vi "dfd_DFXP Add (ss).vi"(5 "quantize output? (T)":bool=TRUE, 7 "op params":T5={"source"=0, "is floating?"=FALSE, "o-mode"=enum."Wrap", "q-mode"=enum."Truncation", "wl"=1, "high limit"=0, "low limit"=0, "iwl"=0, "sign?"=TRUE} {"source" items=["Coef a/k"=0, "Coef b/v"=7, "Input"=1, "Output"=2, "Multiplicand"=3, "Product"=4, "Sum"=5, "Delay"=6, "Gain"=8]}, 8 "filtering statistics in":T4(array[cluster]) {"statistics information"."min value" format="%.2f"; "statistics information"."max value" format="%.2f"; "Quantizer Source" items=["Coefficients a/k"=0, "Coefficients b/v"=7, "Input"=1, "Output"=2, "Multiplicand"=3, "Product"=4, "Sum"=5, "Delay"=6]}, 9 "Value in 2":T1={"value"=0, "wl"=0, "iwl"=0, "Signed"=TRUE} {"value" format="%.0x"}, 11 "Value in":T1={"value"=0, "wl"=0, "iwl"=0, "Signed"=TRUE} {"value" format="%.0x"}) -> (0 "filtering statistics out":T4(array[cluster]) {"statistics information"."min value" format="%.2f"; "statistics information"."max value" format="%.2f"; "Quantizer Source" items=["Coefficients a/k"=0, "Coefficients b/v"=7, "Input"=1, "Output"=2, "Multiplicand"=3, "Product"=4, "Sum"=5, "Delay"=6]}, 3 "Value out":T1={"value"=0, "wl"=0, "iwl"=0, "Signed"=TRUE} {"value" format="%.0x"})   [LabVIEW 2017, in "NI_DigFilter_FXP.lvlib"]
uses:
  <vilib>/addons/Digital Filter Design/NI_DigFilter_FXP.lvlib
  <vilib>/addons/Digital Filter Design/_Objects.llb/dfd_DFXP Data Type (scaler).ctl
  <vilib>/addons/Digital Filter Design/_Objects.llb/dfd_DFXP Data Type 128bits (scaler).ctl
  <vilib>/addons/Digital Filter Design/_Objects.llb/dfd_DFXP Operation Parameter.ctl
  <vilib>/addons/Digital Filter Design/_Objects.llb/dfd_Internal Quantization Srcs.ctl
  <vilib>/addons/Digital Filter Design/_Objects.llb/DFD Quantization Sources.ctl
  <vilib>/addons/Digital Filter Design/_Objects.llb/DFD FXP Statistics Data.ctl
  <vilib>/addons/Digital Filter Design/NI_DigFilterLicensed.lvlib
panel:
  in  "Value type64":T1={"value"=0, "wl"=0, "iwl"=0, "Signed"=TRUE} {"value" format="%.0x"}
  in  "Value type":T1={"value"=0, "wl"=0, "iwl"=0, "Signed"=TRUE} {"value" format="%.0x"}
  in  "Value type":T7 {"Low 64" format="%.0x"; "High 64" format="%.0x"}
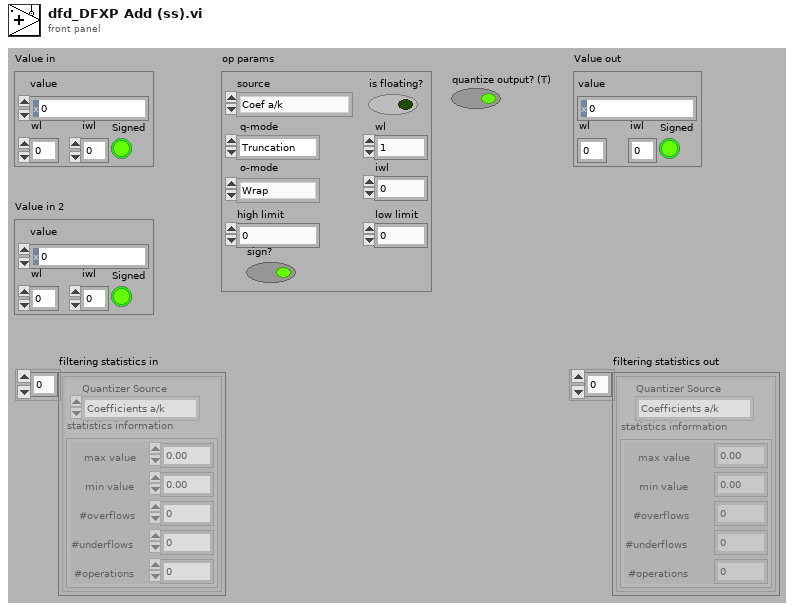
[diagram p1: front panel]
types:
  T1 = typedef "dfd_DFXP Data Type (scaler).ctl" = cluster{"value":i64, "wl":i16, "iwl":i16, "Signed":bool}
  T2 = typedef "NI_DigFilterLicensed.lvlib/DFD Quantization Sources.ctl" = u16
  T3 = typedef "NI_DigFilterLicensed.lvlib/DFD FXP Statistics Data.ctl" = cluster{"max value":ext, "min value":ext, "#overflows":i32, "#underflows":i32, "#operations":i32}
  T4 = cluster{"Quantizer Source":T2, "statistics information":T3}[]
  T5 = typedef "dfd_DFXP Operation Parameter.ctl" = cluster{"source":T6, "is floating?":bool, "o-mode":enum16{"Saturation", "Wrap"}, "q-mode":enum16{"Nearest", "Truncation"}, "wl":i16, "high limit":i64, "low limit":i64, "iwl":i16, "sign?":bool}
  T6 = typedef "NI_DigFilterLicensed.lvlib/dfd_Internal Quantization Srcs.ctl" = u16
  T7 = typedef "dfd_DFXP Data Type 128bits (scaler).ctl" = cluster{"Low 64":u64, "High 64":i64, "wl":i16, "iwl":i16}
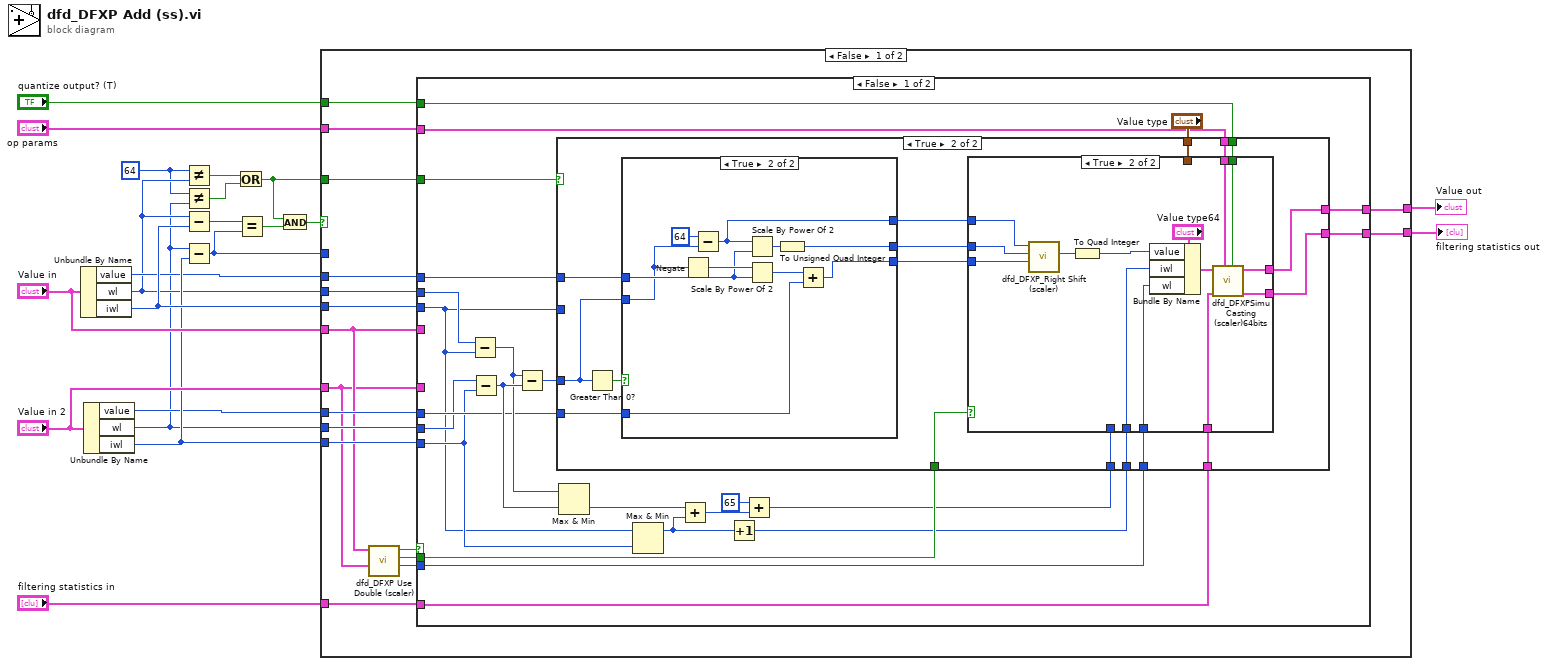
[diagram p0: block diagram]
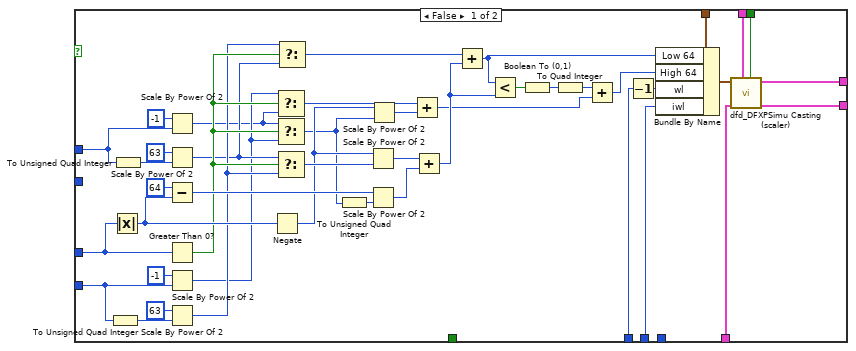
[diagram p2: hidden frame]
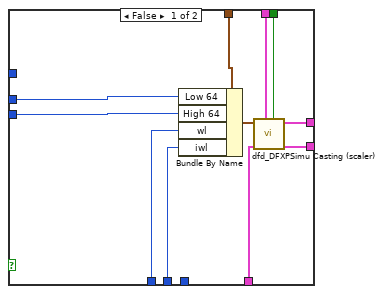
[diagram p3: hidden frame]
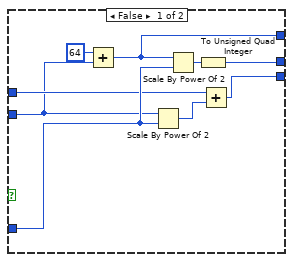
[diagram p4: hidden frame]
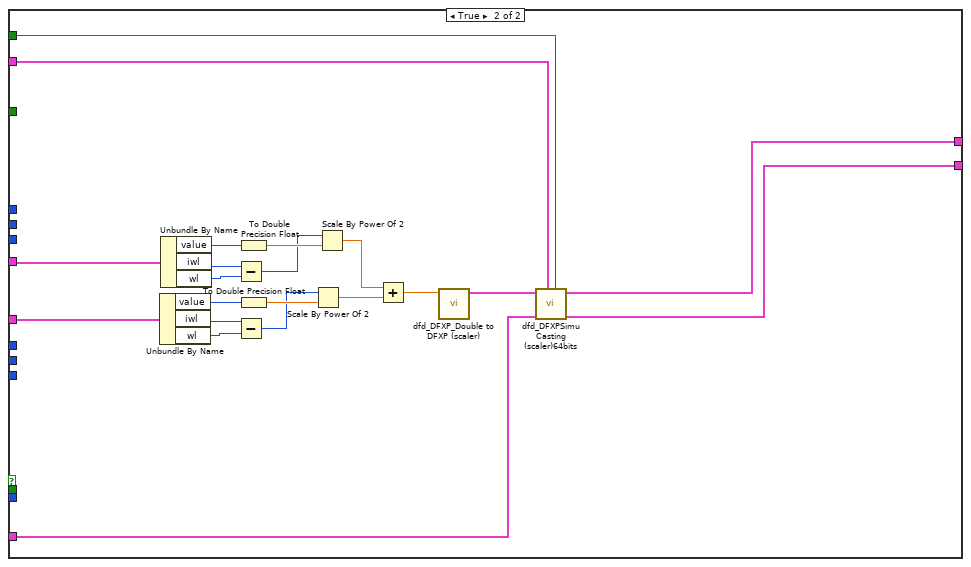
[diagram p5: hidden frame]
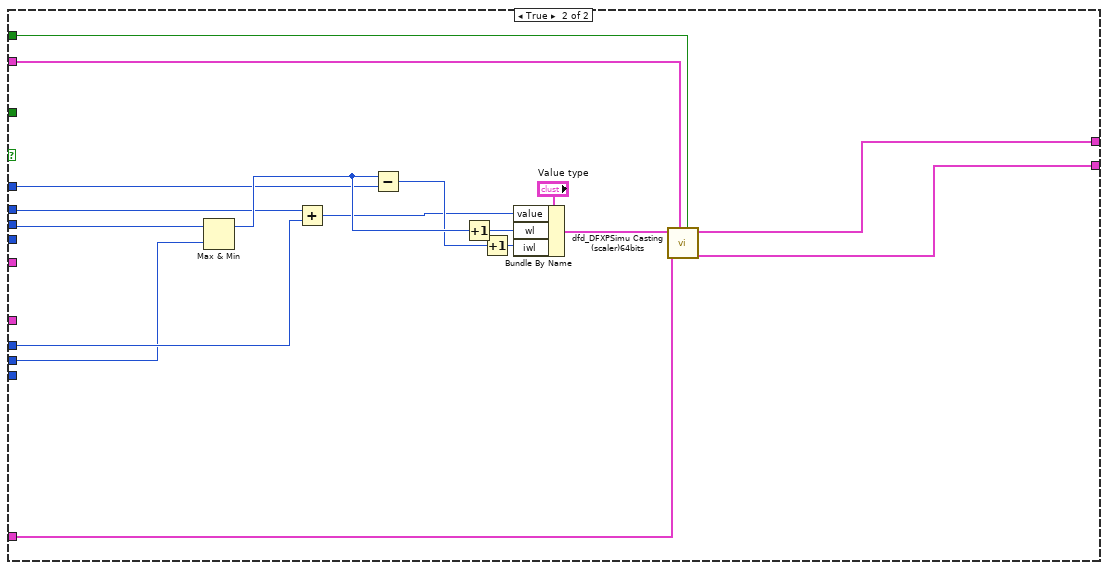
[diagram p6: hidden frame]
diagram:
  w3 = i16 64 ("y")
  n1 = Unbundle By Name("Value in") -> ("value"=w12:i64, "wl"=w5:i16, "iwl"=w16:i16)
  n2 = Unbundle By Name("Value in 2") -> ("value"=w11:i64, "wl"=w4:i16, "iwl"=w15:i16)
  n3 = Not Equal?(x=w3, y=w5) -> (x != y?=w6:bool)
  n4 = Not Equal?(x=w3, y=w4) -> (x != y?=w2:bool)
  n5 = Subtract(x=w5, y=w16) -> (x-y=w10:i16)
  n6 = Subtract(x=w4, y=w15) -> (x-y=w9:i16)
  n7 = Or(x=w6, y=w2) -> (x .or. y?=w1:bool)
  n8 = Equal?(x=w10, y=w9) -> (x = y?=w8:bool)
  n9 = And(x=w1, y=w8) -> (x .and. y?=w7:bool)
  n10 = case shown="False" w7 {
    tunnel: w5 -> [w35 w193]
    tunnel: w16 -> [w34 _]
    tunnel: w4 -> [w32 w191]
    tunnel: w15 -> [w31 _]
    tunnel: w11 -> [w33 w192]
    tunnel: w12 -> [w36 w194]
    tunnel: "Value in" -> [w26 _]
    tunnel: "Value in 2" -> [w25 _]
    tunnel: "filtering statistics in" -> [w30 w190]
    tunnel: "op params" -> [w37 w196]
    tunnel: [w28 w188] -> w18
    tunnel: [w29 w189] -> w19
    tunnel: "quantize output? (T)" -> [w38 w197]
    tunnel: w9 -> [_ w195]
    tunnel: w1 -> [w27 _]
    frame False {
      n11 = call <vilib>:"dfd_DFXP Use Double (scaler).vi"("Value in 2"=w25, "Value in"=w26) -> ("Result wl"=w22:i16, "Use 64?"=w23:bool, "Use double?"=w24:bool)  [unwired: 7 out]
      n12 = case shown="False" w24 {
        tunnel: [w45 w183] -> w28
        tunnel: w30 -> [w46 w185]
        tunnel: [w44 w184] -> w29
        tunnel: w37 -> [w43 w182]
        tunnel: w36 -> [w56 _]
        tunnel: w35 -> [w55 _]
        tunnel: w34 -> [w39 _]
        tunnel: w33 -> [w54 _]
        tunnel: w32 -> [w53 _]
        tunnel: w31 -> [w52 _]
        tunnel: w38 -> [w42 w181]
        tunnel: w26 -> [_ w177]
        tunnel: w25 -> [_ w172]
        tunnel: w27 -> [w51 _]
        tunnel: w23 -> [w50 _]
        tunnel: w22 -> [w40 _]
        frame False {
          n13 = Subtract(x=w55, y=w39) -> (x-y=w58:i16)
          n14 = Subtract(x=w53, y=w52) -> (x-y=w62:i16)
          n15 = Subtract(x=w58, y=w62) -> (x-y=w41:i16)
          n16 = Max & Min(x=w58, y=w62) -> (min(x,y)=w61:i16)  [unwired: 1 out]
          n17 = Max & Min(x=w39, y=w52) -> (max(x,y)=w57:i16)  [unwired: 1 out]
          n18 = Add(x=w61, y=w57) -> (x+y=w60:i16)
          n19 = Increment(x=w57) -> (x+1=w47:i16)
          n20 = Add(x=i16 65, y=w60) -> (x+y=w48:i16)
          n21 = case shown="True" w51 {
            tunnel: w41 -> [w76 w119]
            tunnel: w56 -> [w75 w121]
            tunnel: w54 -> [w77 w120]
            tunnel: w50 -> [_ w116]
            tunnel: "Value type" -> [w69 w115]
            tunnel: w48 -> [w71 w114]
            tunnel: w47 -> [w70 w113]
            tunnel: w46 -> [w68 w112]
            tunnel: [w64 w111] -> w45
            tunnel: [w65 w110] -> w44
            tunnel: w43 -> [w67 w109]
            tunnel: w42 -> [w66 w108]
            tunnel: w40 -> [_ w106]
            tunnel: w39 -> [_ _]
            frame False {
              n22 = To Unsigned Quad Integer(1:w77) -> (0:w100:u64)
              n23 = Absolute Value(x=w76) -> (abs(x)=w97:i16)
              n24 = To Unsigned Quad Integer(1:w75) -> (0:w101:u64)
              n25 = Scale By Power Of 2(n=-1, x=w75) -> (x*2^n=w78:i64)
              n26 = Scale By Power Of 2(n=63, x=w101) -> (x*2^n=w89:u64)
              n27 = Subtract(x=i16 64, y=w97) -> (x-y=w104:i16)
              n28 = Greater Than 0?(x=w76) -> (x > 0?=w91:bool)
              n29 = Scale By Power Of 2(n=-1, x=w77) -> (x*2^n=w79:i64)
              n30 = Scale By Power Of 2(n=63, x=w100) -> (x*2^n=w90:u64)
              n31 = Negate(x=w97) -> (-x=w94:i16)
              n32 = Select(t=w79, s=w91, f=w78) -> (s? t:f=w87:i64)
              n33 = Select(t=w78, s=w91, f=w79) -> (s? t:f=w92:i64)
              n34 = Select(t=w89, s=w91, f=w90) -> (s? t:f=w95:u64)
              n35 = Select(t=w90, s=w91, f=w89) -> (s? t:f=w86:u64)
              n36 = To Unsigned Quad Integer(1:w92) -> (0:w96:u64)
              n37 = Scale By Power Of 2(n=w94, x=w95) -> (x*2^n=w80:u64)
              n38 = Scale By Power Of 2(n=w104, x=w96) -> (x*2^n=w93:u64)
              n39 = Scale By Power Of 2(n=w94, x=w92) -> (x*2^n=w88:i64)
              n40 = Add(x=w87, y=w88) -> (x+y=w82:i64)
              n41 = Add(x=w80, y=w93) -> (x+y=w85:u64)
              n42 = Add(x=w86, y=w85) -> (x+y=w73:u64)
              n43 = Less?(x=w73, y=w85) -> (x < y?=w84:bool)
              n44 = Boolean To (0,1)(Boolean=w84) -> (0, 1=w83:i16)
              n45 = To Quad Integer(1:w83) -> (0:w81:i64)
              n46 = Add(x=w81, y=w82) -> (x+y=w72:i64)
              n47 = Decrement(x=w71) -> (x-1=w63:i16)
              n48 = Bundle By Name(cluster=w69, "Low 64"=w73, "High 64"=w72, "wl"=w63, "iwl"=w70) -> (w74:T7)
              n49 = call <vilib>:"dfd_DFXPSimu Casting (scaler).vi"("quantize output? (T)"=w66, "op params"=w67, "filtering statistics in"=w68, "Value in"=w74) -> ("filtering statistics out"=w64:T4, "Value out"=w65:T1)  [unwired: 6 out]
            }
            frame True {
              n50 = Greater Than 0?(x=w119) -> (x > 0?=w122:bool)
              n51 = case shown="True" w122 {
                tunnel: [w151 w161] -> w118
                tunnel: [w150 w158] -> w117
                tunnel: w121 -> [w152 w163]
                tunnel: w120 -> [w154 w159]
                tunnel: w119 -> [w149 w162]
                tunnel: [w148 w157] -> w107
                frame False {
                  n52 = Add(x=i16 64 ("y"), y=w149) -> (x+y=w148:i16)
                  n53 = Scale By Power Of 2(n=w149, x=w154) -> (x*2^n=w153:i64)
                  n54 = Scale By Power Of 2(n=w148, x=w154) -> (x*2^n=w155:i64)
                  n55 = To Unsigned Quad Integer(1:w155) -> (0:w151:u64)
                  n56 = Add(x=w152, y=w153) -> (x+y=w150:i64)
                }
                frame True {
                  n57 = Negate(x=w162) -> (-x=w165:i16)
                  n58 = Subtract(x=i16 64 ("y"), y=w162) -> (x-y=w157:i16)
                  n59 = Scale By Power Of 2(n=w157, x=w163) -> (x*2^n=w164:i64)
                  n60 = Scale By Power Of 2(n=w165, x=w163) -> (x*2^n=w160:i64)
                  n61 = To Unsigned Quad Integer(1:w164) -> (0:w161:u64)
                  n62 = Add(x=w160, y=w159) -> (x+y=w158:i64)
                }
              }
              n63 = case shown="True" w116 {
                tunnel: w118 -> [w131 w146]
                tunnel: w117 -> [w130 w145]
                tunnel: w115 -> [w132 _]
                tunnel: w114 -> [w129 _]
                tunnel: w113 -> [w128 w140]
                tunnel: w112 -> [w127 w138]
                tunnel: [w126 w136] -> w111
                tunnel: [w125 w135] -> w110
                tunnel: w109 -> [w124 w144]
                tunnel: w108 -> [w123 w134]
                tunnel: w107 -> [_ w147]
                tunnel: w106 -> [_ w139]
                frame False {
                  n64 = Bundle By Name(cluster=w132, "Low 64"=w131, "High 64"=w130, "wl"=w129, "iwl"=w128) -> (w133:T7)
                  n65 = call <vilib>:"dfd_DFXPSimu Casting (scaler).vi"("quantize output? (T)"=w123, "op params"=w124, "filtering statistics in"=w127, "Value in"=w133) -> ("filtering statistics out"=w126:T4, "Value out"=w125:T1)  [unwired: 6 out]
                }
                frame True {
                  n66 = call <vilib>:"dfd_DFXP_Right Shift (scaler).vi"("High 64"=w145, "Low 64"=w146, "Num"=w147) -> ("Low 64"=w142:u64)  [unwired: 8 out]
                  n67 = To Quad Integer(1:w142) -> (0:w141:i64)
                  n68 = Bundle By Name(cluster="Value type64", "value"=w141, "iwl"=w140, "wl"=w139) -> (w137:T1)
                  n69 = call <vilib>:"dfd_DFXPSimu Casting (scaler)64bits.vi"("quantize output?(T)"=w134, "op params"=w144, "filtering statistics in"=w138, "Value in"=w137) -> ("filtering statistics out"=w136:T4, "Value out"=w135:T1)  [unwired: 6 out]
                }
              }
            }
          }
        }
        frame True {
          n70 = Unbundle By Name(w172) -> ("value"=w174:i64, "iwl"=w170:i16, "wl"=w171:i16)
          n71 = Unbundle By Name(w177) -> ("value"=w179:i64, "iwl"=w168:i16, "wl"=w167:i16)
          n72 = Subtract(x=w168, y=w167) -> (x-y=w178:i16)
          n73 = Subtract(x=w170, y=w171) -> (x-y=w173:i16)
          n74 = To Double Precision Float(number=w179) -> (double precision float=w180:dbl)
          n75 = To Double Precision Float(number=w174) -> (double precision float=w175:dbl)
          n76 = Scale By Power Of 2(n=w173, x=w175) -> (x*2^n=w169:dbl)
          n77 = Scale By Power Of 2(n=w178, x=w180) -> (x*2^n=w176:dbl)
          n78 = Add(x=w176, y=w169) -> (x+y=w187:dbl)
          n79 = call <vilib>:"dfd_DFXP_Double to DFXP (scaler).vi"("Double"=w187) -> ("FXP"=w186:T1)  [unwired: 10 out]
          n80 = call <vilib>:"dfd_DFXPSimu Casting (scaler)64bits.vi"("quantize output?(T)"=w181, "op params"=w182, "filtering statistics in"=w185, "Value in"=w186) -> ("filtering statistics out"=w183:T4, "Value out"=w184:T1)  [unwired: 6 out]
        }
      }
    }
    frame True {
      n81 = Max & Min(x=w193, y=w191) -> (max(x,y)=w203:i16)  [unwired: 1 out]
      n82 = Add(x=w194, y=w192) -> (x+y=w199:i64)
      n83 = Subtract(x=w203, y=w195) -> (x-y=w202:i16)
      n84 = Increment(x=w203) -> (x+1=w200:i16)
      n85 = Increment(x=w202) -> (x+1=w201:i16)
      n86 = Bundle By Name(cluster="Value type", "value"=w199, "wl"=w200, "iwl"=w201) -> (w198:T1)
      n87 = call <vilib>:"dfd_DFXPSimu Casting (scaler)64bits.vi"("quantize output?(T)"=w197, "op params"=w196, "filtering statistics in"=w190, "Value in"=w198) -> ("filtering statistics out"=w188:T4, "Value out"=w189:T1)  [unwired: 6 out]
    }
  }
  "Value out" <- w19
  "filtering statistics out" <- w18
